vi "SDI Close Device.vi"(10 "DevIndex":i32, 11 "DevType":i32) -> (3 "function return":i32)   [LabVIEW 2010, in "ControlSDI.lvlib"]
doc: "int WINAPI SDI_CloseDevice(int DevType,int DevIndex);"
uses:
  ControlSDI.lvlib
  ControlSDI/Ginkgo_Driver.dll
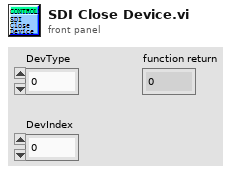
[diagram p1: front panel]
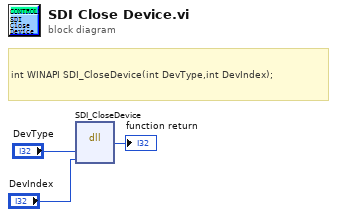
[diagram p0: block diagram]
diagram:
  # "int WINAPI SDI_CloseDevice(int DevType,int DevIndex);"
  n1 = dll-call lib="E:/Project/vt_ginkgo/truck/Ginkgo Driver/vs2010/Ginkgo_USB-I2C&SPI&CAN_API_v2.0.3.3/lib/labview_32bit/ControlSDI/Ginkgo_Driver.*" fn="SDI_CloseDevice"("DevType"="DevType", "DevIndex"="DevIndex") -> (→"function return":i32)  [unwired: 5 in, 2 out]
